vi "dataAcq_bufferVIServer.vi"(0 "reference":refnum<class "OSA.lvclass">, 1 "interferogram prop set":T1 {"peakToPeak position (cm)" format="%.2f"; "peakToPeak, (counts)" format="%.2f"; "X max (cm)" format="%.2f"; "X min (cm)" format="%.2f"}, 2 "action":T4(ring), 3 "bufferSize spectrum":i32, 4 "bufferSize interferogram":i32, 5 "error in (no error)":errorcluster, 6 "interferogram set":sgl[](array[numeric]) format="%.2f", 7 "spectrum set Y":sgl[](array[numeric]) format="%.2f", 9 "spectrum prop set":T3) -> (11 "spectrum X":sgl[](array[numeric]) format="%.2f", 12 "interferogram":sgl[](array[numeric]) format="%.2f", 13 "spectrum Y":sgl[](array[numeric]) format="%.2f", 14 "duplicate reference":refnum<class "OSA.lvclass">, 15 "interferogram prop set":T1 {"peakToPeak position (cm)" format="%.2f"; "peakToPeak, (counts)" format="%.2f"; "X max (cm)" format="%.2f"; "X min (cm)" format="%.2f"}, 16 "timed out":bool, 18 "spectrum property":T3, 19 "error out":errorcluster)   [LabVIEW 2010, in "OSA.lvclass"]
doc: "Latest retrieved data, (interferogram or spectrum), stored in this buffer vi."
uses:
  OSA.lvclass
  typeDef/xVal_option.ctl
panel:
  in  "spectrum set X":sgl[](array[numeric]) format="%.2f"
  in  "VI Refnum":refnum<vi>
  # "data per spectrometer \narranged in columns, (second index)"
  # "only Y data saved, (no X data created during sampling),\nto keep allocated data memory as small as possible."
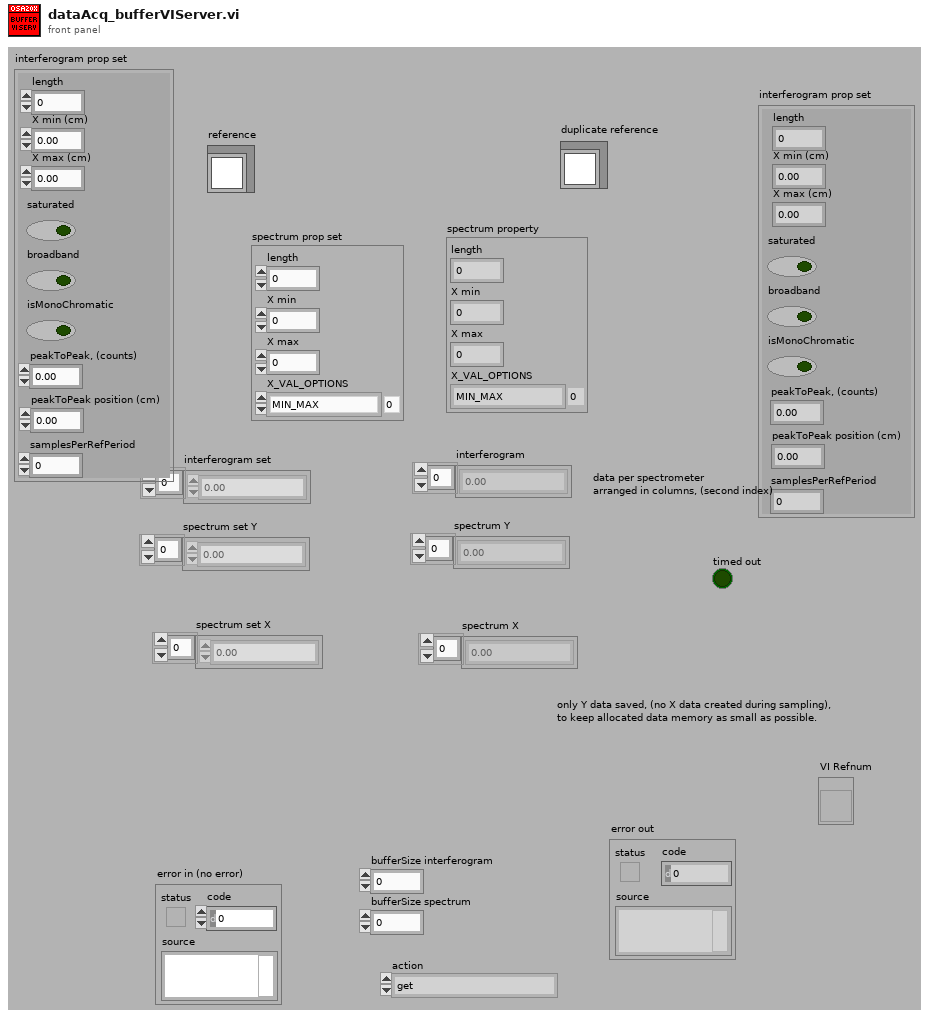
[diagram p1: front panel]
types:
  T1 = cluster{"length":u32, "X min (cm)":sgl, "X max (cm)":sgl, "saturated":bool, "broadband":bool, "isMonoChromatic":bool, "peakToPeak, (counts)":dbl, "peakToPeak position (cm)":dbl, "samplesPerRefPeriod":i32}
  T2 = typedef "OSA.lvclass/xVal_option.ctl" = enum16{"MIN_MAX", "ARRAY"}
  T3 = cluster{"length":u32, "X min":sgl, "X max":sgl, "X_VAL_OPTIONS":T2}
  T4 = enum16{"get", "init", "set interferogram", "set spectrum", "cleanUp"}
  T5 = typedef "OSA.lvclass/ObjectAttributes.ctl" = cluster{"Stop":bool, "dataType":T6, "spectrometerIdx":u16, "buffer size interferogram":i32, "interferogram":cluster{"new":bool, "plot_x_ min":sgl, "plot_x_max":sgl, "plot_y_min":sgl, "plot_y_max":sgl, "Graph Intrfrgrm":T7, "timeStamp":u32, "signal (%)":dbl, "traces":cluster{"idx":u32, "broadBand":bool, "monoChromatic":bool, "peakToPeakSignal":dbl, "peakToPeakPos":dbl}[], "traces idx last":i32}, "spectrum":cluster{"new":bool, "plot_x_min":sgl, "plot_x_max":sgl, "plot_unit_x":T8, "plot_unit_y":T9, "plot_y_min":sgl, "plot_y_max":sgl, "Graph Spectrum":T7, "timeStamp":u32, "X_VAL_OPTIONS":enum16{"MIN_MAX", "ARRAY"}, "traces":cluster{"idx":u32}[], "traces idx last":i32}, "Thorlabs_OSA_64.lvclass:queue_action.ctlqueue ref":refnum<queue>, "action":T10, "plot zoom step":dbl, "buffer semaphore":T11, "acq stopped":bool, "dataType active":T6, "temperature (degr C)":sgl, "pressure (hPa)":sgl, "rel humidity (%)":sgl, "settings":cluster{"resolution":T12, "sensitivity":T13, "Average":bool, "average nr":u32, "apodisation":T14, "acq delay (ms)":u32, "airMesure":T15, "wmtr on":bool, "intfgrm_smooth_width":u16, "intfgrm_smooth_nrOfPasses":u16, "intfgrm_smooth":T16, "phaseCorrection":T17, "zeroFill":u8, "spectr_smooth":T16, "spectr_smooth_width":u16, "spectr_smooth_nrOfPasses":u16, "resolution (/cm)":sgl, "REF wavelength, (nm)":dbl, "gain_idx":u16, "gainAuto":bool, "gain_relative":dbl, "PD sensitivity mode":T18, "PD senseMode implemented":bool, "SensorTemperature implemented":bool, "SensorPressure implemented":bool, "SensorHumidity implemented":bool}, "peaks position":sgl[], "peaks width":sgl[], "peaks height":sgl[], "peaks max nr":u32, "peaks latest nr":i32, "peaks new":bool, "power":dbl, "power new":bool, "path":string, "wavelength (WNr)":dbl, "wavelength new":bool, "buffer size spectrum":i32, "status":string, "VI reference":refnum<vi>, "funcPointer":u64, "libraryPointer":u64, "singleAcquisition":bool, "coherenceLength (cm)":dbl, "coherenceLength new":bool, "spectrometer model":string, "spectrometer serial nr":string, "peaks thld left":sgl[], "peaks thld right":sgl[], "coherenceLength error (cm)":dbl, "ADC bits":u16, "peaks position centroid":sgl[], "peaks height centroid":sgl[], "OSA series":T19, "channel index spectrum":u16, "spectrometer rangeLow, (/cm)":dbl, "spectrometer rangeHigh, (/cm)":dbl, "channel index interferogram":u16}
  T6 = typedef "OSA.lvclass/acq_dataType.ctl" = enum16{"none", "interferogram", "spectrum"}
  T7 = typedef "OSA.lvclass/graph_intensity.ctl" = refnum<vi>
  T8 = typedef "OSA.lvclass/spectrum_x_unit.ctl" = enum16{"wavenr/cm", "THz", "eV", "nm_air", "nm_vac"}
  T9 = typedef "OSA.lvclass/y_unit.ctl" = enum16{"ADC counts", "dBm pwr absolute", "dBm pwr density", "mW pwr absolute", "mW pwr density"}
  T10 = typedef "OSA.lvclass/queue_action.ctl" = enum16{"none", "stop", "GUI_plotInterferogram", "GUI_plotSpectrum", "GUI_plotInterferogramRescale", "GUI_plotSpectrumRescale", "GUI_plotInterferogramReset", "GUI_plotSpectrumReset", "GUI_plotInterferogramAutoScaleY", "GUI_plotSpectrumAutoScaleY", "GUI_plotInterferogramZoomOut", "GUI_plotSpectrumZoomOut", "GUI_plotInterferogramPane", "GUI_plotSpectrumPane", "GUI_plotInterferogramZoomMouse", "GUI_plotSpectrumZoomMouse", "ENVIRONMENT temperature", "ENVIRONMENT pressure", "MODE_resolution set", "MODE_resolution get", "MODE_sensitivity set", "MODE_sensitivity get", "MODE_PDTemperature set", "MODE_PDTemperature get", "REBOOT/RESET firmware", "ACQASYNC_acquireSingleSpectrum", "ACQASYNC_continuous start", "ACQASYNC_continuous stop\n", "ACQASYNC_get last interferogram", "ACQASYNC_get last spectrum", "ACQASYNC_get last waveNr", "ACQOPT_interferogram smoothing set", "ACQOPT_interferogram smoothing get", "ACQOPT_spectrum smoothing set", "ACQOPT_spectrum smoothing get", "ACQOPT_apodisation type set", "ACQOPT_apodisation type get", "ACQOPT_phase correction type set", "ACQOPT_phase correction type get", "ACQOPT_acqIntervall_set", "ACQOPT_acqIntervall_get", "ACQOPT_average spectrum set", "ACQOPT_average spectrum get", "ACQOPT_rolling average set", "ACQOPT_rolling average get", "ACQOPT_zero fill factor set", "ACQOPT_zero fill factor get", "ACQOPT_cycle counting set", "ACQOPT_cycle counting get", "ACQOPT_air measure option set", "ACQOPT_air measure option get", "ACQOPT_gainLevel auto get", "ACQOPT_gainLevel auto set", "ACQOPT_gainLevel get", "ACQOPT_gainLevel set", "ACQOPT_getAll", "INSTRUMENT_PROPERTY_range_WaveNr_min", "INSTRUMENT_PROPERTY_range_WaveNr_max", "INSTRUMENT_PROPERTY_reference_wavelength_cm^-1", "INSTRUMENT_PROPERTY_samplesPerRefPeriod", "INSTRUMENT_PROPERTY_resolution_waveNrPercm", "INSTRUMENT_PROPERTY_availableGainLevels", "INSTRUMENT_PROPERTY_status", "CONVERT", "ANALYSE_POWER", "ANALYSE_PEAKS", "ANALYSE_WAVELENGTH", "ANALYSE_SPECTRUM", "ANALYSE_INTERFEROGRAM", "ANALYSE_COHERENCE_LENGTH", "MATH", "MATH_power", "MATH_peaks", "FILE", "miscellaneous"}
  T11 = typedef "Semaphore RefNum" = refnum<k1>
  T12 = typedef "OSA.lvclass/resolution.ctl" = enum16{"low", "high"}
  T13 = typedef "OSA.lvclass/sensitivityMode.ctl" = enum16{"low", "low medium", "high medium", "high"}
  T14 = typedef "OSA.lvclass/apodisation.ctl" = enum16{"NONE", "NORTON_BEER_WEAK", "NORTON_BEER_MEDIUM", "NORTON_BEER_STRONG", "TRIANGULAR", "COSINE", "HANN", "HAMMING", "BLACKMANHARRIS3", "BLACKMANHARRIS4", "GAUSSIAN"}
  T15 = typedef "OSA.lvclass/airMeasure.ctl" = enum16{"TEMPERATURE", "PRESSURE"}
  T16 = typedef "OSA20X_misc.lvlib/interferogram_smoothing.ctl" = enum16{"NONE", "BINOMIAL", "SAVITSKY_GOLAY", "FOURIER", "MOVING_AVERAGE", "GAUSSIAN"}
  T17 = typedef "OSA.lvclass/phaseCorrection.ctl" = enum16{"NONE", "MERTZ", "FORMAN", "MERTZ_FILE", "FORMAN_FILE", "FUTURE COMP."}
  T18 = typedef "OSA20X_misc.lvlib/PDTemperatureMode.ctl" = enum16{"cool: better sensitivity/noise floor", "warm: extended wl range"}
  T19 = typedef "OSA.lvclass/OSA_series.ctl" = enum16{"OSA200", "OSA300", "UNKNOWN"}
  T20 = typedef "OSA20X.lvclass/xVal_option.ctl" = enum16{"MIN_MAX", "ARRAY"}
  T21 = cluster{"length":u32, "X min":sgl, "X max":sgl, "X_VAL_OPTIONS":T20}
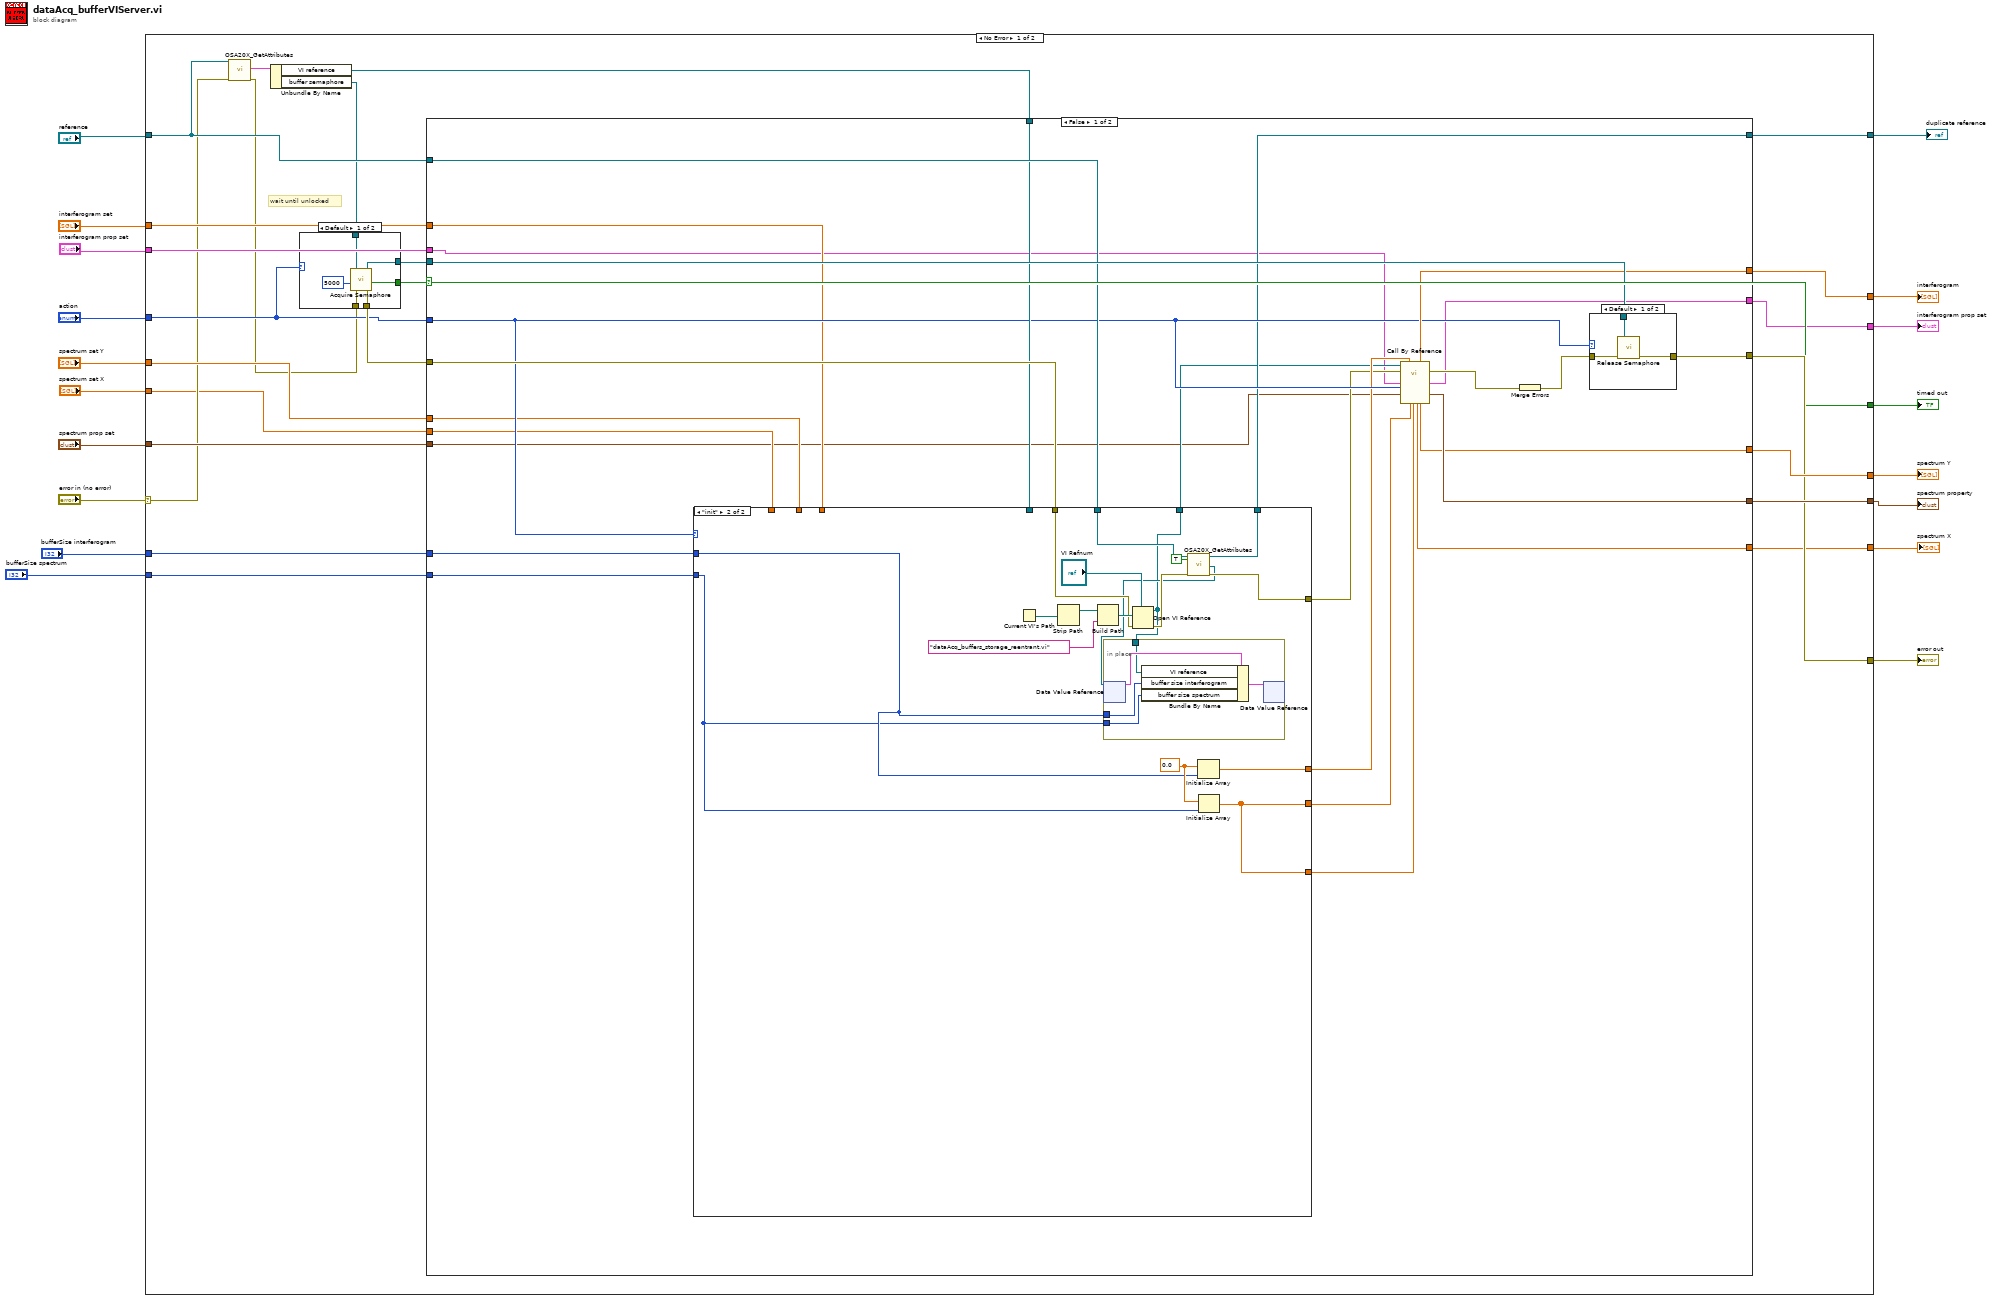
[diagram p0: block diagram]
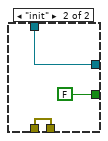
[diagram p2: hidden frame]
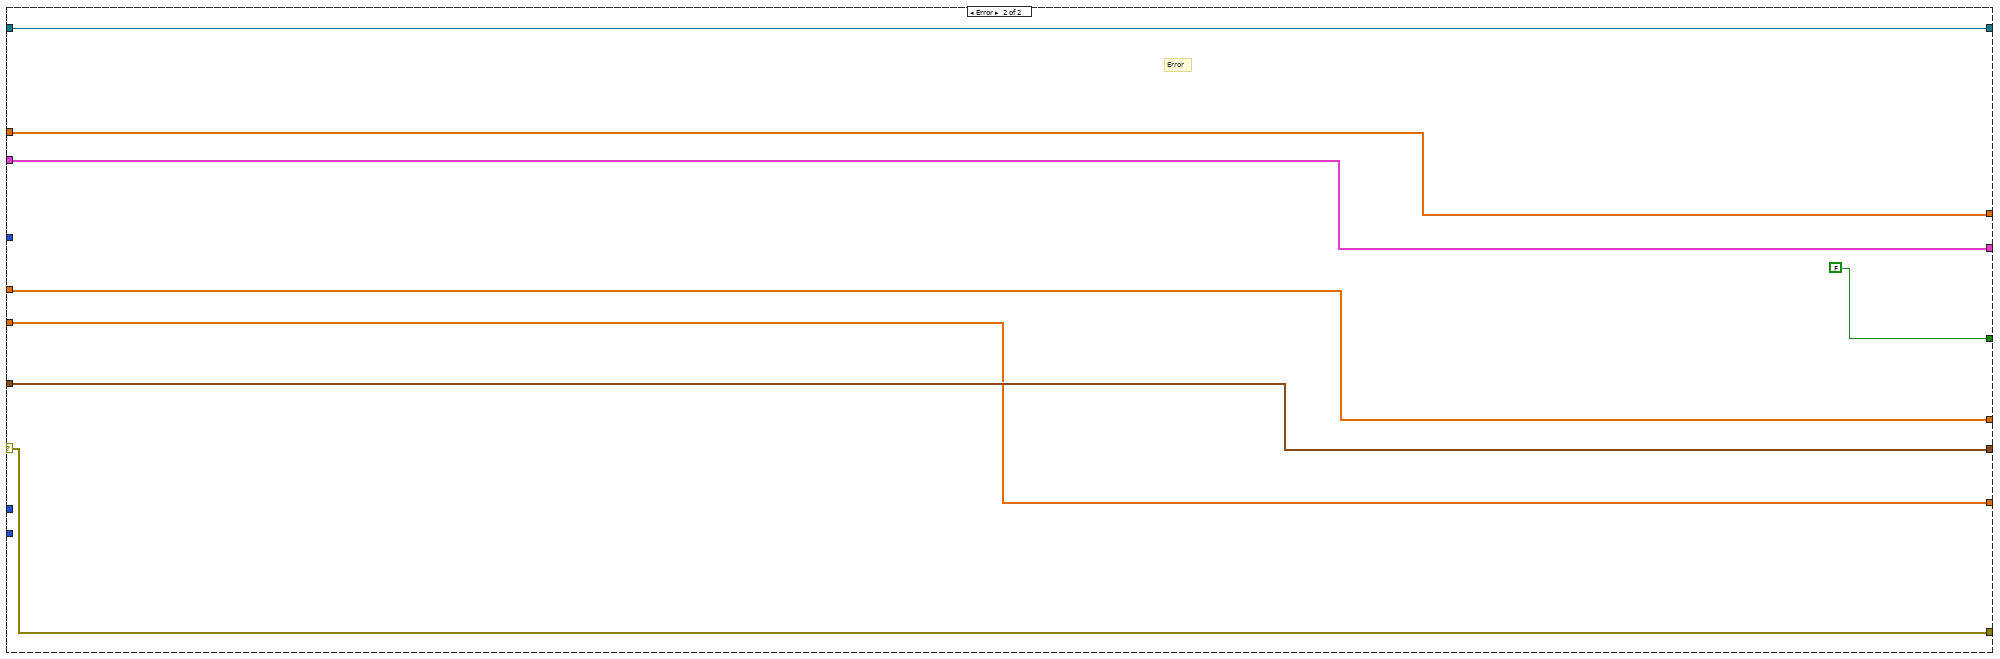
[diagram p6: hidden frame]
diagram:
  n1 = case shown="No Error" "error in (no error)" {
    selector: "error in (no error)" -> [w25 w124]
    tunnel: [w30 w124] -> w18
    tunnel: "reference" -> [w26 w125]
    tunnel: [w36 w125] -> w15
    tunnel: "action" -> [w27 _]
    tunnel: "interferogram set" -> [w38 w123]
    tunnel: "interferogram prop set" -> [w37 w122]
    tunnel: "spectrum set Y" -> [w32 w121]
    tunnel: "spectrum prop set" -> [w31 w120]
    tunnel: [w35 w123] -> w10
    tunnel: [w28 w122] -> w9
    tunnel: [w33 w121] -> w8
    tunnel: [w34 w120] -> w7
    tunnel: "bufferSize interferogram" -> [w40 _]
    tunnel: [w29 FALSE ("timed out")] -> w5
    tunnel: "bufferSize spectrum" -> [w39 _]
    tunnel: [w20 w118] -> w2
    tunnel: "spectrum set X" -> [w19 w118]
    frame No Error {
      # "wait until unlocked"
      n2 = call "OSA20X_GetAttributes.vi"("reference in"=w26, "error in (no error)"=w25) -> ("Data"=w21:T5, "error out"=w24:errorcluster)  [unwired: 14 in, 2 out]
      n3 = Unbundle By Name(w21) -> ("VI reference"=w22:refnum<vi>, "buffer semaphore"=w23:T11)
      n4 = case shown="Default" w27 {
        tunnel: [w47 w51] -> w42
        tunnel: w24 -> [w46 w49]
        tunnel: [w45 w49] -> w41
        tunnel: [w44 FALSE ("timed out")] -> w29
        tunnel: w23 -> [w43 w51]
        frame Default {
          n5 = call <vilib>:"Acquire Semaphore.vi"("error in (no error)"=w46, "ms timeout (-1)"=5000, "semaphore"=w43) -> ("error out"=w45:errorcluster, "timed out"=w44:bool, "semaphore out"=w47:T11)  [unwired: 2 in]
        }
        frame "init" {
        }
      }
      n6 = case shown="False" w29 {
        tunnel: [w72 w116] -> w35
        tunnel: [w57 w114] -> w28
        tunnel: [w71 w112] -> w33
        tunnel: w41 -> [w74 w117]
        tunnel: [w77 w117] -> w30
        tunnel: w42 -> [w76 _]
        tunnel: w26 -> [w75 w115]
        tunnel: w40 -> [w63 _]
        tunnel: w39 -> [w62 _]
        tunnel: w38 -> [w65 w116]
        tunnel: w37 -> [w58 w114]
        tunnel: [w60 w115] -> w36
        tunnel: [w73 w113] -> w34
        tunnel: w32 -> [w64 w112]
        tunnel: w31 -> [w52 w113]
        tunnel: w27 -> [w67 _]
        tunnel: w22 -> [w68 _]
        tunnel: [w54 w111] -> w20
        tunnel: w19 -> [w53 w111]
        frame False {
          n7 = case shown="\"init\"" w67 {
            tunnel: [w83 w91] -> w59
            tunnel: w75 -> [w87 w98]
            tunnel: w74 -> [w86 w100]
            tunnel: [w86 w97] -> w61
            tunnel: [w87 w96] -> w60
            tunnel: w68 -> [w83 _]
            tunnel: [w85 w94] -> w66
            tunnel: w65 -> [w85 _]
            tunnel: w64 -> [w84 _]
            tunnel: [w84 w88] -> w56
            tunnel: w63 -> [_ w90]
            tunnel: w62 -> [_ w89]
            tunnel: [w82 w88] -> w55
            tunnel: w53 -> [w82 _]
            frame Default {
            }
            frame "init" {
              w95 = sgl 0.0 ("Numeric")
              n8 = Current VI's Path() -> (path=w101:path)
              n9 = Strip Path(path=w101) -> (stripped path=w104:path)  [unwired: 1 out]
              n10 = Build Path(base path=w104, name or relative path="dataAcq_buffers_storage_reentrant.vi" ("machine name (\"\":  open local reference)")) -> (appended path=w102:path)
              n11 = Open VI Reference(type specifier VI Refnum (for type only)="VI Refnum", vi path=w102, error in (no error)=w100) -> (vi reference=w91:refnum<vi>, error out=w99:errorcluster)  [unwired: 3 in]
              n12 = call "OSA20X_GetAttributes.vi"("reference in"=w98, "OnlyGetDvrReference(False)"=TRUE, "error in (no error)"=w99) -> ("reference out"=w96:refnum<class "OSA.lvclass">, "DataRef"=w92:refnum<data-value>, "error out"=w97:errorcluster)  [unwired: 13 in, 1 out]
              n13 = in-place {
                in-place-border: w91 -> [w109]
                in-place-border: w90 -> [w108]
                in-place-border: w89 -> [w107]
                n14 = in-place-dvr #1(w92) -> (w110:T5)  [unwired: 1 out]
                n15 = Bundle By Name(cluster=w110, "VI reference"=w109, "buffer size interferogram"=w108, "buffer size spectrum"=w107) -> (w106:T5)
                n16 = in-place-dvr #1(w106) -> ()  [unwired: 2 out]
              }
              n17 = Initialize Array(w95, w90) -> (w94:sgl[])
              n18 = Initialize Array(w95, w89) -> (w88:sgl[])
            }
          }
          n19 = call-by-ref "?"(reference=w59, error in=w61, "interferogram prop set"=w58, "action"=w67, "spectrum prop set"=w52, "interferogram set"=w66, "spectrum set Y"=w56, "spectrum set X"=w55) -> (error out=w70:errorcluster, "spectrum X"=w54:sgl[], "interferogram"=w72:sgl[], "spectrum Y"=w71:sgl[], "interferogram prop set"=w57:T1, "spectrum property"=w73:T21)  [unwired: 9 in, 1 out]
          n20 = Merge Errors(w70) -> (w69:errorcluster)
          n21 = case shown="Default" w67 {
            tunnel: [w80 w81] -> w77
            tunnel: w76 -> [w79 _]
            tunnel: w69 -> [w78 w81]
            frame Default {
              n22 = call <vilib>:"Release Semaphore.vi"("error in (no error)"=w78, "semaphore"=w79) -> ("error out"=w80:errorcluster)  [unwired: 4 in, 1 out]
            }
            frame "init" {
            }
          }
        }
        frame True {
        }
      }
    }
    frame Error {
      # "Error"
    }
  }
  "error out" <- w18
  "duplicate reference" <- w15
  "interferogram" <- w10
  "interferogram prop set" <- w9
  "spectrum Y" <- w8
  "spectrum property" <- w7
  "timed out" <- w5
  "spectrum X" <- w2
